vi "Add String Separator.vi"(10 "separator":string="; ", 11 "string in":string) -> (3 "string out":string)   [LabVIEW 2020, in "Measurement Plugin Session Management V1.lvlib" / "Session Reservation.lvclass"]
uses:
  Session Reservation.lvclass
  Session Reservation.lvclass/Session Reservation.ctl
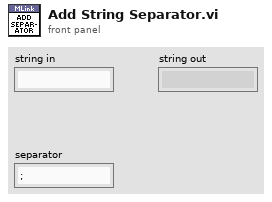
[diagram p1: front panel]
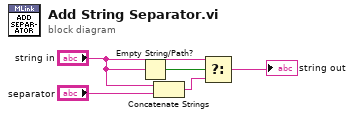
[diagram p0: block diagram]
diagram:
  n1 = Empty String/Path?(string/path="string in") -> (empty?=w1:bool)
  n2 = Concatenate Strings("string in", "separator") -> (w3:string)
  n3 = Select(t="string in", s=w1, f=w3) -> (s? t:f=→"string out":string)
